vi "AO_Create.vi"(0 "reference in":refnum<class "AO.lvclass">, 5 "error in (no error)":errorcluster) -> (14 "reference out":refnum<class "AO.lvclass">, 19 "error out":errorcluster)   [LabVIEW 2019, in "AO.lvclass"]
doc: "Constructor."
uses:
  AO.lvclass
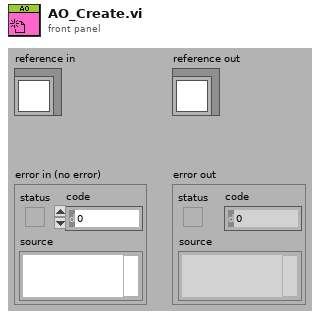
[diagram p1: front panel]
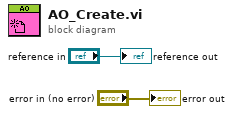
[diagram p0: block diagram]
diagram:
  "error out" <- "error in (no error)"
  "reference out" <- "reference in"
